vi "Refactor Msg.vi"() -> ()   [LabVIEW 2021]
panel:
  in  "Refactor":bool
  in  "Rename (optional)":string
  in  "Msgs":string(combo)
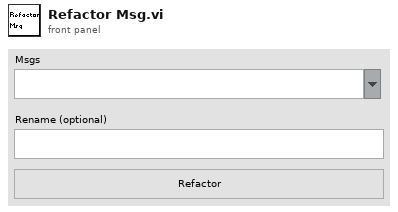
[diagram p1: front panel]
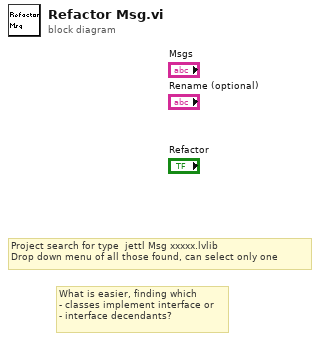
[diagram p0: block diagram]
diagram:
  # "What is easier, finding which\n- classes implement interface or\n- interface decendants?"
  # "Project search for type  jettl Msg xxxxx.lvlib \nDrop down menu of all those found, can select only one"
